vi "SeriellWriteFPGA_ECD.vi"   [LabVIEW 2017]
uses:
  <vilib>/rvi/Emulation/niFpgaGetClockAttributes.vi
  <vilib>/rvi/Emulation/niFpgaSctlEmulationGetInTimedLoop.vi
  <vilib>/rvi/Emulation/niFpgaEmulationReportErrorSimple.vi
  GVglobalStopFPGA_ECD.vi
  <vilib>/rvi/DataTransferAndStorage/Container/Common/niFpgaContainerExecOnDevCompGetState.vi
  <vilib>/rvi/Emulation/niFpgaEmulationIsFPGAContextNoSignature.vi
  <vilib>/rvi/errors/niFpgaSetErrorForExecOnDevCompSimple.vi
  <vilib>/rvi/eio/common/nirviEmuReportErrorAndStop.vi
  <vilib>/rvi/DataTransferAndStorage/Container/Common/niFpgaContainerGetUniqueNameForEmu.vi
  <vilib>/rvi/FIFO/Fifo_Resource/nirvififoEmulationSetSize.vi
  <vilib>/rvi/FIFO/Fifo_Resource/nirviFifoEmulationQueueMgr.vi
  <instcachedir>/0/nirviFifoEmulationQueueMgr_E5CAEC123FF24DC58D834DCA3CDAA9B5.lvgen/nirviFifoEmulationQueueMgr_E5CAEC123FF24DC58D834DCA3CDAA9B5_002.vi
  <vilib>/rvi/FIFO/Fifo_Resource/nirvififoEmulationDetermineInputValidOut.vi
  <vilib>/rvi/FIFO/Fifo_Resource/nirvififoEmulationCreateLock.vi
  <vilib>/rvi/Emulation/niFpgaProcessEmulError.vi
  <vilib>/rvi/FIFO/Fifo_Resource/nirvififoEmulationObtainLock.vi
  <vilib>/rvi/FIFO/Fifo_Resource/nirvififoEmulationReleaseLock.vi
  <vilib>/rvi/occurrence/nirviWaitOnOccurrenceBase.vi
  <vilib>/rvi/errors/nirviReportUnexpectedCaseInternalError.vi
  <vilib>/rvi/errors/nirviReportUnexpectedCaseInternalError (U32).vi
  <vilib>/Utility/error.llb/Clear Errors.vi
  <vilib>/rvi/interface/RandomDataEmulation/niFpgaRandomDataHandleErrors.vi
  <vilib>/rvi/eio/common/nirviEmuTemplateMethod_errors.vi
  <vilib>/rvi/Emulation/niFpgaCriticalErrorInLSC.vi
  <vilib>/rvi/DataTransferAndStorage/Container/XNode/niFpgaContainer.xnode
  <vilib>/rvi/FIFO/Fifo_Resource/niFpgaFifoEmulationRefIn.vi
  <vilib>/eio/EIOMethodNode/EIOMethodNode.xnode
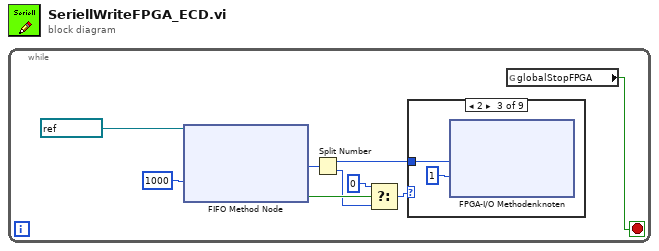
[diagram p0: block diagram]
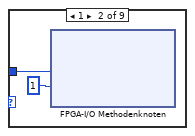
[diagram p3: hidden frame]
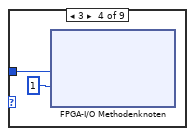
[diagram p4: hidden frame]
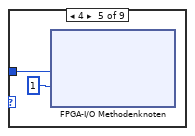
[diagram p5: hidden frame]
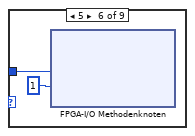
[diagram p6: hidden frame]
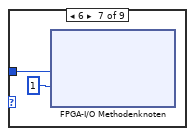
[diagram p7: hidden frame]
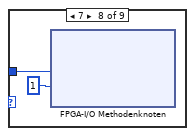
[diagram p8: hidden frame]
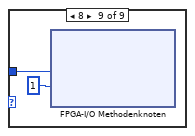
[diagram p9: hidden frame]
diagram:
  n1 = while {
    stop <- w9 stop-if-true
    n2 = xnode ("FIFO Method Node")("Timeout"=1000, "FIFO (Eingang)"=refnum<k21> "WRITE") -> ("Element"=w4:u16, "Timeout?"=w7:bool)  [unwired: 1 out]
    n3 = Split Number(x=w4) -> (hi(x)=w2:u8, lo(x)=w3:u8)
    n4 = Select(t=u8 0, s=w7, f=w3) -> (s? t:f=w6:u8)
    n5 = case shown="2" w6 {
      tunnel: w2 -> [_ w11 w13 w15 w17 w19 w21 w23 w25]
      frame 0, Default {
      }
      frame 1 {
        n6 = xnode "FPGA-I/O Methodenknoten"("Data"=w11, "Timeout (ms)"=1) -> ()  [unwired: 1 in, 2 out]
      }
      frame 2 {
        n7 = xnode "FPGA-I/O Methodenknoten"("Data"=w13, "Timeout (ms)"=1) -> ()  [unwired: 1 in, 2 out]
      }
      frame 3 {
        n8 = xnode "FPGA-I/O Methodenknoten"("Data"=w15, "Timeout (ms)"=1) -> ()  [unwired: 1 in, 2 out]
      }
      frame 4 {
        n9 = xnode "FPGA-I/O Methodenknoten"("Data"=w17, "Timeout (ms)"=1) -> ()  [unwired: 1 in, 2 out]
      }
      frame 5 {
        n10 = xnode "FPGA-I/O Methodenknoten"("Data"=w19, "Timeout (ms)"=1) -> ()  [unwired: 1 in, 2 out]
      }
      frame 6 {
        n11 = xnode "FPGA-I/O Methodenknoten"("Data"=w21, "Timeout (ms)"=1) -> ()  [unwired: 1 in, 2 out]
      }
      frame 7 {
        n12 = xnode "FPGA-I/O Methodenknoten"("Data"=w23, "Timeout (ms)"=1) -> ()  [unwired: 1 in, 2 out]
      }
      frame 8 {
        n13 = xnode "FPGA-I/O Methodenknoten"("Data"=w25, "Timeout (ms)"=1) -> ()  [unwired: 1 in, 2 out]
      }
    }
    n14 = global read "GVglobalStopFPGA_ECD.vi" "globalStopFPGA"() -> (w9:bool)
  }
